vi "Gas Select Lock Check.vi"(8 "error in":errorcluster, 9 "Software Rev":u8, 10 "Volumetric Units Code":i32, 11 "Mass Units Code":i32) -> (0 "error out":errorcluster, 2 "Lock Gas Select":bool)   [LabVIEW 2018]
doc: "Determines if a firmware revision 5 or lower device allows gas selection changes or not. Older devices (firmware revision 5 and lower) made the conversion to true mass flow rate using a constant density factor, and did not allow selectable gases."
panel:
  # "This is a VI to lock out the ability to select different gases if the unit \nis configured for true mass and has a software revision older than 6v00\n\nThis is necessary because a true mass unit on current software performs \nthe calculation to true mass after the mass flow rate is determined, and \nis locked to a specific density factor. Altering the gas selected will not \nautomatically alter the density, leaving the mass conversion incorrect."
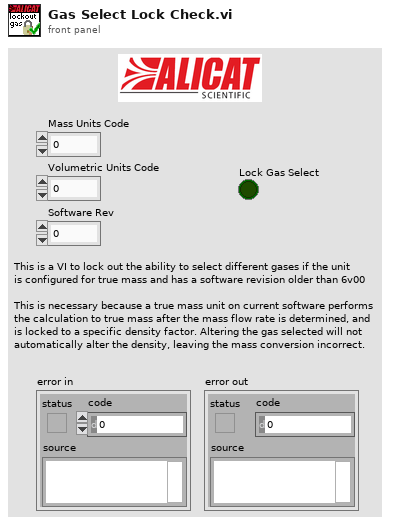
[diagram p1: front panel]
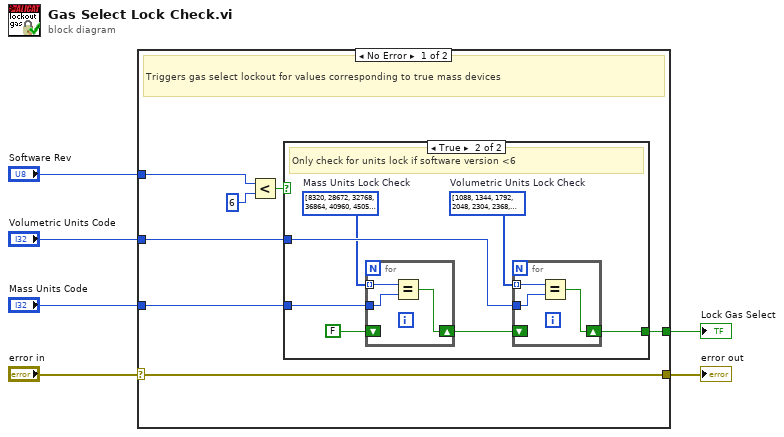
[diagram p0: block diagram]
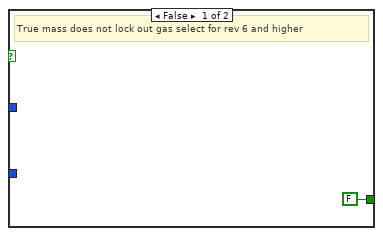
[diagram p2: hidden frame]
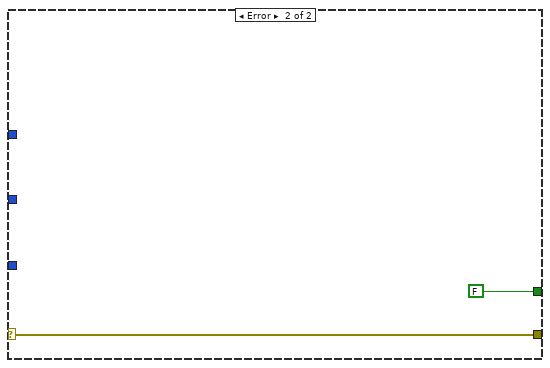
[diagram p3: hidden frame]
diagram:
  n1 = case shown="No Error" "error in" {
    selector: "error in" -> [w10 w28]
    tunnel: "Volumetric Units Code" -> [w13 _]
    tunnel: "Mass Units Code" -> [w12 _]
    tunnel: [w11 FALSE] -> w4
    tunnel: [w10 w28] -> w2
    tunnel: "Software Rev" -> [w7 _]
    frame No Error {
      # "Triggers gas select lockout for values corresponding to true mass devices"
      n2 = Less?(x=w7, y=u8 6) -> (x < y?=w8:bool)
      n3 = case shown="True" w8 {
        tunnel: w13 -> [_ w20]
        tunnel: w12 -> [_ w18]
        tunnel: [FALSE w17] -> w11
        frame False {
          # "True mass does not lock out gas select for rev 6 and higher"
        }
        frame True {
          w19 = i32[] [8320, 28672, 32768, 36864, 40960, 45056, 49152, 53248, 53376]  # Mass Units Lock Check
          w21 = i32[] [1088, 1344, 1792, 2048, 2304, 2368, 2560, 2816, 3072, 3584]  # Volumetric Units Lock Check
          # "Only check for units lock if software version <6"
          n4 = for {
            tunnel: w19 -> [w24] mode=indexing
            tunnel: w18 -> [w23]
            shift-right: [w22] -> w15
            shift-left: FALSE -> [_]
            n5 = Equal?(x=w24, y=w23) -> (x = y?=w22:bool)
          }
          n6 = for {
            tunnel: w21 -> [w27] mode=indexing
            tunnel: w20 -> [w26]
            shift-right: [w25] -> w17
            shift-left: w15 -> [_]
            n7 = Equal?(x=w27, y=w26) -> (x = y?=w25:bool)
          }
        }
      }
    }
    frame Error {
    }
  }
  "Lock Gas Select" <- w4
  "error out" <- w2
